vi "Remove Typedefs from Variant.vi"(8 "错误输入":errorcluster, 10 "Variant with typedefs":variant) -> (0 "错误输出":errorcluster, 2 "Variant without typedef":variant)   [LabVIEW 2012, in "TD Tools.lvlib"]
uses:
  TD Tools.lvlib
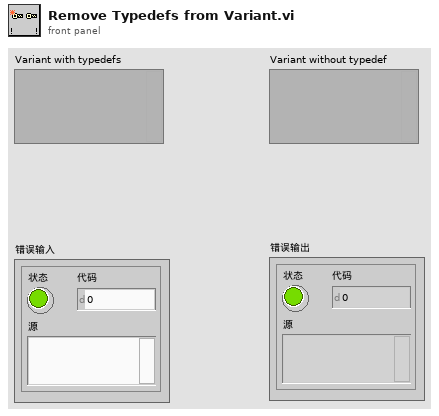
[diagram p1: front panel]
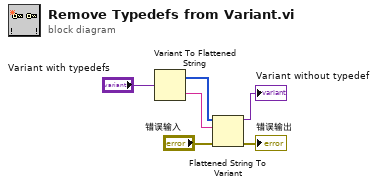
[diagram p0: block diagram]
diagram:
  n1 = Variant To Flattened String(Variant="Variant with typedefs") -> (data string=w4:string, 1:w5:i16[])
  n2 = Flattened String To Variant(4:"错误输入", 6:w4, 7:w5) -> (0:→"错误输出":errorcluster, 3:→"Variant without typedef":variant)
